vi "addMessageToQueue.vi"(8 "error in (no error)":errorcluster, 10 "message":string, 11 "TCPCommunicator in":refnum<class "TCPCommunicator.lvclass">) -> (0 "error out":errorcluster, 2 "timed out?":bool, 3 "TCPCommunicator out":refnum<class "TCPCommunicator.lvclass">)   [LabVIEW 2016, in "TCPCommunicator.lvclass"]
uses:
  TCPCommunicator.lvclass
  TCPCommunicator.lvclass/TCPCommunicator.ctl
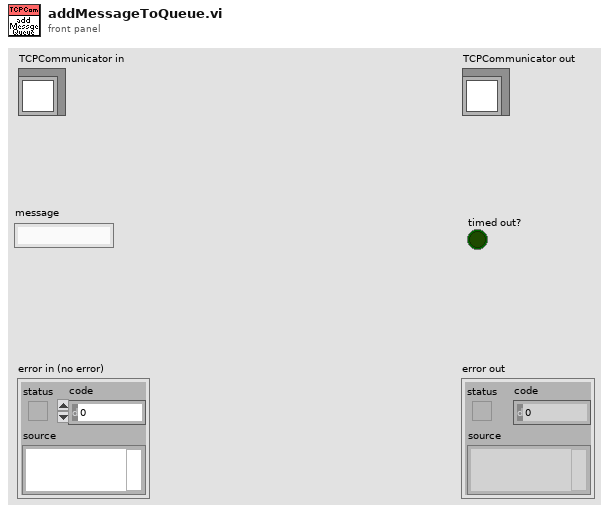
[diagram p1: front panel]
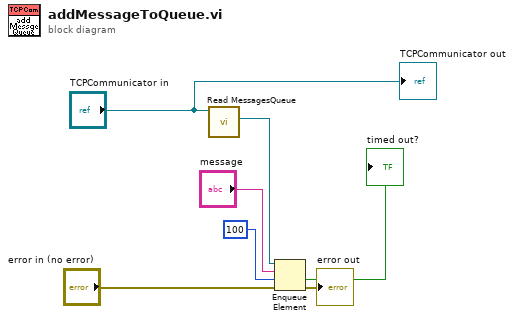
[diagram p0: block diagram]
diagram:
  n1 = call "Read MessagesQueue.vi"("TCPCommunicator in"="TCPCommunicator in") -> ("MessagesQueue"=w6:refnum<queue>)  [unwired: 8 in, 2 out]
  n2 = Enqueue Element(queue=w6, element="message", timeout in ms (-1)=100, error in (no error)="error in (no error)") -> (timed out?=→"timed out?":bool, error out=→"error out":errorcluster)  [unwired: 1 out]
  "TCPCommunicator out" <- "TCPCommunicator in"
